vi "Actor Core.vi"(8 "error in":errorcluster, 11 "Logger in":refnum<class "Logger.lvclass">) -> (0 "error out":errorcluster, 3 "Actor out":refnum<class "Actor.lvclass">)   [LabVIEW 2015, in "Logger Actor.lvlib" / "Logger.lvclass"]
doc: "(<B>Filename</B>: Actor Framework.lvlib:Actor.lvclass:Actor Core.vi)\n\nReceives messages to the actor, reacts to them, and initiates any error handling that may shut the actor down.\n\nDescendant classes may override this VI to append parallel tasks for the actor to complete while it handles messages. Overrides use the Call Parent Method node."
uses:
  Logger.lvclass
  <vilib>/ActorFramework/Actor/Actor.lvclass
  Logger.lvclass/Logger.ctl
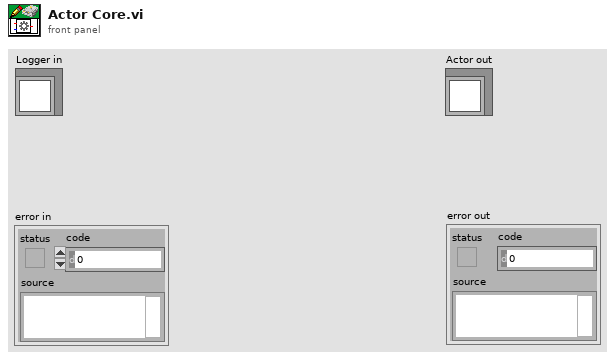
[diagram p1: front panel]
types:
  T1 = enum16{"open", "open or create", "create or replace", "create", "open (read-only)"}
  T2 = enum16{"big-endian, network order", "native, host order", "little-endian"}
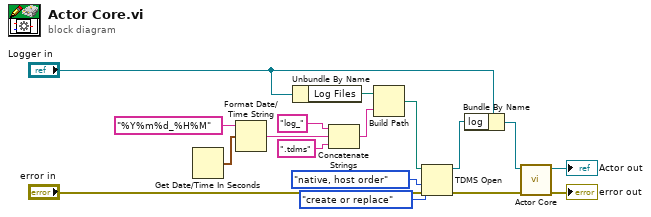
[diagram p0: block diagram]
diagram:
  n1 = Get Date/Time In Seconds() -> (seconds since 1Jan1904=w9:timestamp)
  n2 = Format Date/Time String(time format string (%c)="%Y%m%d_%H%M", seconds (now)=w9) -> (date/time string=w6:string)  [unwired: 1 in]
  n3 = Unbundle By Name("Logger in") -> ("Log Files"=w11:path)
  n4 = Concatenate Strings("log_" ("string"), w6, ".tdms" ("string")) -> (w4:string)
  n5 = Build Path(base path=w11, name or relative path=w4) -> (appended path=w3:path)
  n6 = TDMS Open(8:"error in", 9:T2."native, host order" ("byte order (2:little-endian)"), 10:T1."create or replace" ("operation (0:open)"), 11:w3) -> (0:w13:errorcluster, 3:w2:refnum<k34>)  [unwired: 3 in]
  n7 = Bundle By Name(cluster="Logger in", "log"=w2) -> (w14:refnum<class "Logger.lvclass">)
  n8 = call-parent "Actor Core.vi"("error in"=w13, "Actor in"=w14) -> ("error out"=→"error out":errorcluster, "Actor out"=→"Actor out":refnum<class "Actor.lvclass">)  [unwired: 8 in]
